vi "execute.vi"(8 "error in (no error)":errorcluster, 10 "Context in":refnum<class "Context.lvclass">, 11 "ExitControlCommand in":refnum<class "ExitControlCommand.lvclass">) -> (0 "error out":errorcluster, 2 "Context out":refnum<class "Context.lvclass">, 3 "ExitControlCommand out":refnum<class "ExitControlCommand.lvclass">)   [LabVIEW 2016, in "ExitControlCommand.lvclass"]
uses:
  ExitControlCommand.lvclass
  Context/Context/Context.lvclass
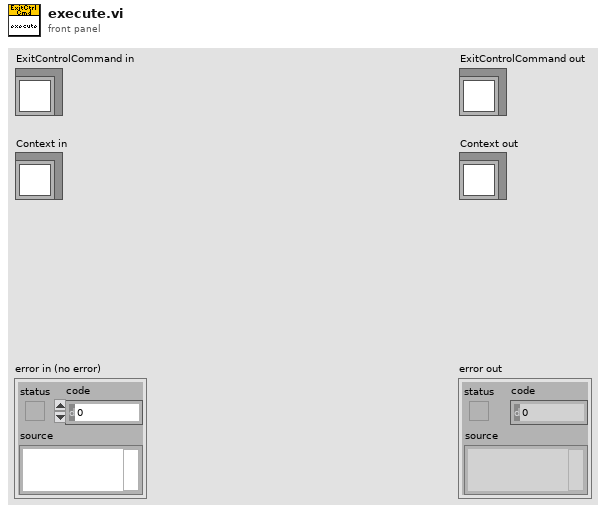
[diagram p1: front panel]
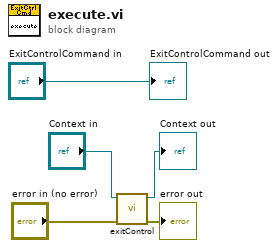
[diagram p0: block diagram]
diagram:
  n1 = call-dynamic "exitControl.vi"("error in (no error)"="error in (no error)", "Context in"="Context in") -> ("error out"=→"error out":errorcluster, "Context out"=→"Context out":refnum<class "Context.lvclass">)  [unwired: 8 in]
  "ExitControlCommand out" <- "ExitControlCommand in"
